vi "CRYData series to tab-delimited datastring.vi"(0 "delimiter":enum16{"tab", "comma", "space", "other"}(ring), 1 "other delim":string, 2 "Data/Wave(if true=wave)?":bool, 4 "precision":i32=2, 5 "notation":enum16{"sci", "float"}(ring)=enum."float", 6 "indices to save":i16[](array[numeric]), 7 "data series":string[](array[string])) -> (3 "tab-delimited data string":string)   [LabVIEW 2013]
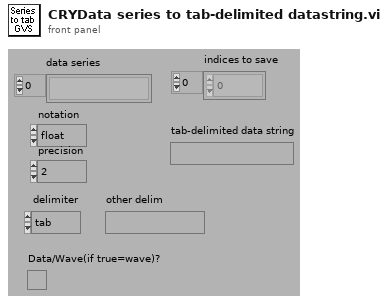
[diagram p1: front panel]
types:
  T1 = typedef "CRYWaveform Cluster.ctl" = cluster{"Waveform":cluster{"X0":dbl, "dX":dbl, "Y":sgl[]}, "X data":u16, "Y data":u16, "Y axis":u16, "X unit":string, "Y unit":string, "Y dB ref":dbl, "display Y":bool, "display X":bool, "Overload?":bool, "Test Info":string, "Step No.":i32, "Name":string, "protected":bool, "Sqc history":string[], "Signal Channel ID":i32, "Plot Settings":cluster{"Color":u32, "Interpolation":u8, "Point Style":u8, "Line Style":u8, "Point Color":u32, "Line Width":u8, "Bar Plot Style":u8, "Fill To":i16}, "AutoProtect":bool}
  T2 = typedef "CRYData Cluster.ctl" = cluster{"Name":string, "Curve":cluster{"x":dbl, "y":dbl, "z":dbl}[], "X data":u16, "Y data":u16, "Z data":u16, "X axis":u16, "Y axis":u16, "Z axis":u16, "X unit":string, "Y unit":string, "Z unit":string, "X dB ref":dbl, "Y dB ref":dbl, "Z dB ref":dbl, "single val":bool, "protected":bool, "display X":bool, "display Y":bool, "display Z":bool, "Test Info":string, "Step No.":i32, "Plot Settings":cluster{"Color":u32, "Interpolation":u8, "Point Style":u8, "Line Style":u8, "Point Color":u32, "Line Width":u8, "Bar Plot Style":u8, "Fill To":i16}, "AutoProtect":bool}
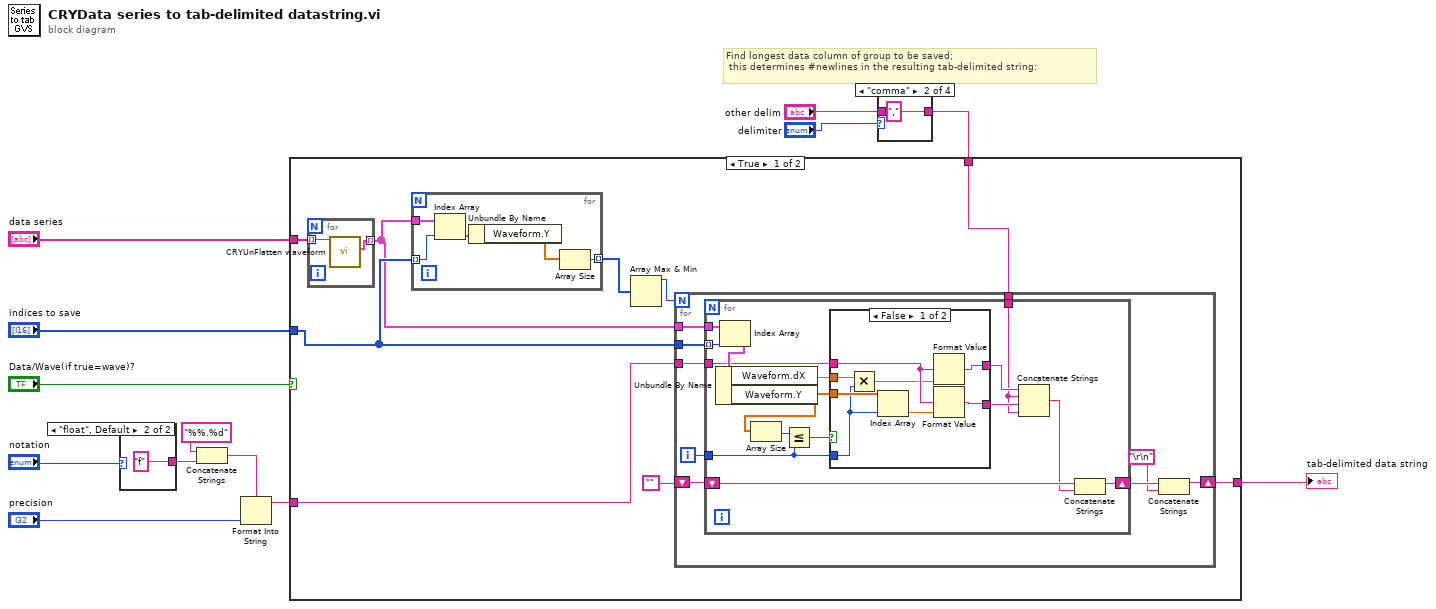
[diagram p0: block diagram]
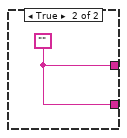
[diagram p2: hidden frame]
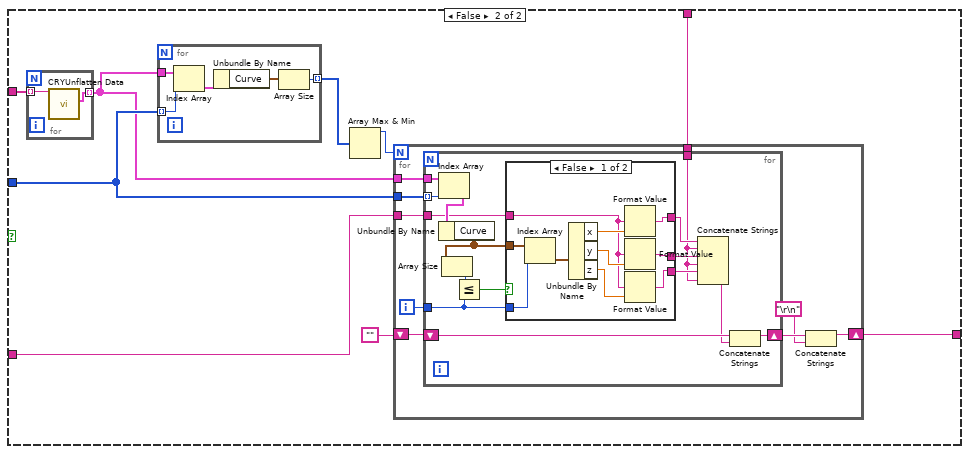
[diagram p3: hidden frame]
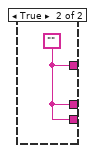
[diagram p4: hidden frame]
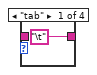
[diagram p5: hidden frame]
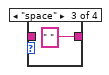
[diagram p6: hidden frame]
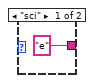
[diagram p8: hidden frame]
diagram:
  # "Find longest data column of group to be saved;\n this determines #newlines in the resulting tab-delimited string:"
  n1 = case shown="\"float\", Default" "notation" {
    tunnel: ["e" "f"] -> w7
    frame "sci" {
    }
    frame "float", Default {
    }
  }
  n2 = Concatenate Strings("%%.%d", w7) -> (w6:string)
  n3 = Format Into String(format string=w6, "precision") -> (resulting string=w5:string)  [unwired: 2 in, 1 out]
  n4 = case shown="\"comma\"" "delimiter" {
    tunnel: "other delim" -> [_ _ _ w19]
    tunnel: ["\t" "," " " w19] -> w2
    frame "tab" {
    }
    frame "comma" {
    }
    frame "space" {
    }
    frame Default {
    }
  }
  n5 = case shown="True" "Data/Wave(if true=wave)?" {
    tunnel: "indices to save" -> [w27 w76]
    tunnel: [w24 w73] -> w12
    tunnel: "data series" -> [w22 w71]
    tunnel: w5 -> [w21 w70]
    tunnel: w2 -> [w20 w69]
    frame True {
      n6 = for {
        tunnel: [w30] -> w23 mode=indexing
        tunnel: w22 -> [w29] mode=indexing
        n7 = call "CRYUnFlatten waveform.vi"("Unflatten Waveform"=w29) -> ("Waveform Cluster"=w30:T1)  [unwired: 8 in, 2 out]
      }
      n8 = for {
        tunnel: w23 -> [w68]
        tunnel: w27 -> [w67] mode=indexing
        tunnel: [w64] -> w28 mode=indexing
        n9 = Index Array(array=w68, index=w67) -> (element=w66:T1)
        n10 = Unbundle By Name(w66) -> ("Waveform.Y"=w65:sgl[])
        n11 = Array Size(array=w65) -> (size(s)=w64:i32)
      }
      n12 = Array Max & Min(array=w28) -> (max value=w26:i32)  [unwired: 3 out]
      n13 = for {
        N: w26 -> [_]
        tunnel: w23 -> [w38]
        tunnel: w27 -> [w39]
        shift-right: [w34] -> w24
        shift-left: "" -> [w36]
        tunnel: w21 -> [w32]
        tunnel: w20 -> [w31]
        i -> [w37]
        n14 = for {
          tunnel: w39 -> [w53] mode=indexing
          tunnel: w38 -> [w54]
          tunnel: w37 -> [w48]
          shift-right: [w43] -> w35
          shift-left: w36 -> [w45]
          tunnel: w32 -> [w42]
          tunnel: w31 -> [w41]
          n15 = Index Array(array=w54, index=w53) -> (element=w50:T1)
          n16 = Unbundle By Name(w50) -> ("Waveform.dX"=w40:dbl, "Waveform.Y"=w49:sgl[])
          n17 = Array Size(array=w49) -> (size(s)=w52:i32)
          n18 = Less Or Equal?(x=w52, y=w48) -> (x <= y?=w51:bool)
          n19 = case shown="False" w51 {
            tunnel: w49 -> [w62 _]
            tunnel: w48 -> [w56 _]
            tunnel: [w61 w63] -> w47
            tunnel: [w60 w63] -> w46
            tunnel: w42 -> [w59 _]
            tunnel: w40 -> [w57 _]
            frame False {
              n20 = Multiply(x=w57, y=w56) -> (x*y=w55:dbl)
              n21 = Index Array(array=w62, index=w56) -> (element=w58:sgl)
              n22 = Format Value(format string=w59, value (0)=w55) -> (output string=w61:string)  [unwired: 1 out]
              n23 = Format Value(format string=w59, value (0)=w58) -> (output string=w60:string)  [unwired: 1 out]
            }
            frame True {
              w63 = ""
            }
          }
          n24 = Concatenate Strings(w47, w41, w46, w41) -> (w44:string)
          n25 = Concatenate Strings(w45, w44) -> (w43:string)
        }
        n26 = Concatenate Strings(w35, "\r\n") -> (w34:string)
      }
    }
    frame False {
      n27 = for {
        tunnel: [w79] -> w72 mode=indexing
        tunnel: w71 -> [w78] mode=indexing
        n28 = call "CRYUnflatten Data.vi"("Unflatten data"=w78) -> ("Datum"=w79:T2)  [unwired: 8 in, 2 out]
      }
      n29 = for {
        tunnel: w72 -> [w119]
        tunnel: w76 -> [w118] mode=indexing
        tunnel: [w115] -> w77 mode=indexing
        n30 = Index Array(array=w119, index=w118) -> (element=w117:T2)
        n31 = Unbundle By Name(w117) -> ("Curve"=w116:cluster{"x":dbl, "y":dbl, "z":dbl}[])
        n32 = Array Size(array=w116) -> (size(s)=w115:i32)
      }
      n33 = Array Max & Min(array=w77) -> (max value=w75:i32)  [unwired: 3 out]
      n34 = for {
        N: w75 -> [_]
        tunnel: w72 -> [w87]
        tunnel: w76 -> [w88]
        shift-right: [w83] -> w73
        shift-left: "" -> [w85]
        tunnel: w70 -> [w81]
        tunnel: w69 -> [w80]
        i -> [w86]
        n35 = for {
          tunnel: w88 -> [w102] mode=indexing
          tunnel: w87 -> [w103]
          tunnel: w86 -> [w97]
          shift-right: [w91] -> w84
          shift-left: w85 -> [w93]
          tunnel: w81 -> [w90]
          tunnel: w80 -> [w89]
          n36 = Index Array(array=w103, index=w102) -> (element=w99:T2)
          n37 = Unbundle By Name(w99) -> ("Curve"=w98:cluster{"x":dbl, "y":dbl, "z":dbl}[])
          n38 = Array Size(array=w98) -> (size(s)=w101:i32)
          n39 = Less Or Equal?(x=w101, y=w97) -> (x <= y?=w100:bool)
          n40 = case shown="False" w100 {
            tunnel: w98 -> [w113 _]
            tunnel: w97 -> [w112 _]
            tunnel: [w107 w114] -> w96
            tunnel: [w106 w114] -> w95
            tunnel: [w105 w114] -> w94
            tunnel: w90 -> [w104 _]
            frame False {
              n41 = Index Array(array=w113, index=w112) -> (element=w111:cluster{"x":dbl, "y":dbl, "z":dbl})
              n42 = Unbundle By Name(w111) -> ("x"=w110:dbl, "y"=w109:dbl, "z"=w108:dbl)
              n43 = Format Value(format string=w104, value (0)=w110) -> (output string=w107:string)  [unwired: 1 out]
              n44 = Format Value(format string=w104, value (0)=w109) -> (output string=w106:string)  [unwired: 1 out]
              n45 = Format Value(format string=w104, value (0)=w108) -> (output string=w105:string)  [unwired: 1 out]
            }
            frame True {
              w114 = ""
            }
          }
          n46 = Concatenate Strings(w96, w89, w95, w89, w94, w89) -> (w92:string)
          n47 = Concatenate Strings(w93, w92) -> (w91:string)
        }
        n48 = Concatenate Strings(w84, "\r\n") -> (w83:string)
      }
    }
  }
  "tab-delimited data string" <- w12
